vi "Computer GPS.vi"() -> ()   [LabVIEW 2009]
uses:
  UDP3-GPS, INS/UDP3rtglob.vi
  <instrlib>/u-blox 5 Series/u-blox 5 Series.lvlib
panel:
  out "output cluster":cluster{"Latitude":dbl, "Longitude":dbl}
  out "Valid Satalites":bool
  in  "stop":bool
  in  "Reset (False)":bool
  in  "VISA resource name":refnum<visa-resource-name>
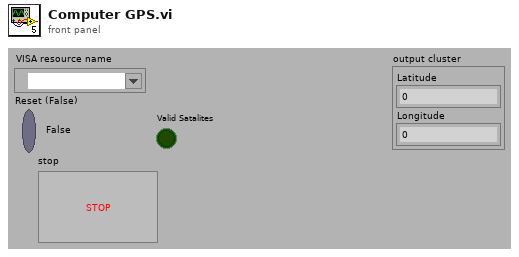
[diagram p1: front panel]
types:
  T1 = cluster{"Timestamp":timestamp, "Latitude":dbl, "Longitude":dbl}[]
  T2 = cluster{"Timestamp":timestamp, "Latitude":dbl, "Longitude":dbl}
  T3 = cluster{cluster{"Latitude":dbl, "Longitude":dbl}, cluster{dbl, dbl, dbl, dbl}}
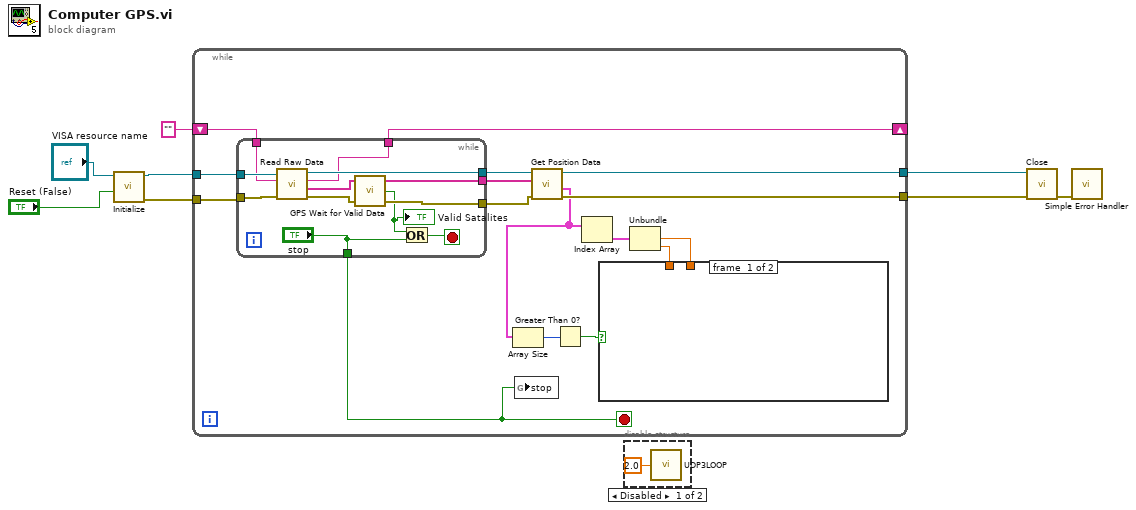
[diagram p0: block diagram]
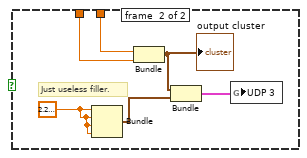
[diagram p3: hidden frame]
diagram:
  n1 = call <instrlib>:"Initialize.vi"("Reset (False)"="Reset (False)", "VISA resource name"="VISA resource name") -> ("error out"=w4:errorcluster, "VISA resource name out"=w5:refnum<visa-resource-name>)  [unwired: 8 in]
  n2 = while {
    shift-right: [w21] -> _
    shift-left: "" ("Remaining Partial Sentence") -> [w24]
    tunnel: w5 -> [w23]
    tunnel: w4 -> [w22]
    tunnel: [w15] -> w2
    tunnel: [w14] -> w3
    stop <- w9 stop-if-true
    n3 = while {
      tunnel: [w42] -> w20
      tunnel: w23 -> [w41]
      tunnel: w22 -> [w40]
      tunnel: w24 -> [w38]
      tunnel: [w35] -> w19
      tunnel: ["stop"] -> w9
      tunnel: [w34] -> w18
      tunnel: [w33] -> w21
      stop <- w39 stop-if-true
      n4 = call <instrlib>:"Read Raw Data.vi"("error in (no error)"=w40, "Previous Partial Sentence"=w38, "VISA resource name"=w41) -> ("error out"=w37:errorcluster, "Complete NMEA Sentences"=w36:string[], "Remaining Partial Sentence"=w33:string, "VISA resource name out"=w42:refnum<visa-resource-name>)  [unwired: 5 in]
      n5 = call "GPS Wait for Valid Data.vi"("error in (no error)"=w37, "Completed NMEA Sentences"=w36) -> ("error out"=w34:errorcluster, "Valid Data"=w32:bool, "Complete NMEA Sentences (Copy)"=w35:string[])  [unwired: 1 in]
      "Valid Satalites" <- w32
      n6 = Or(x=w32, y="stop") -> (x .or. y?=w39:bool)
    }
    n7 = global write "UDP3rtglob.vi" "stop"(w9) -> ()
    n8 = call <instrlib>:"Get Position Data.vi"("error in (no error)"=w18, "Complete NMEA Sentences"=w19, "VISA resource name"=w20) -> ("error out"=w14:errorcluster, "Position Data"=w10:T1, "VISA resource name out"=w15:refnum<visa-resource-name>)  [unwired: 5 in, 1 out]
    n9 = Array Size(array=w10) -> (size(s)=w17:i32)
    n10 = Greater Than 0?(x=w17) -> (x > 0?=w11:bool)
    n11 = Index Array(array=w10) -> (element=w16:T2)  [unwired: 1 in]
    n12 = Unbundle(w16) -> ("Latitude"=w12:dbl, "Longitude"=w13:dbl)  [unwired: 1 out]
    n13 = case shown="True" w11 {
      tunnel: w13 -> [_ w27]
      tunnel: w12 -> [_ w26]
      frame #0 {
      }
      frame #1 {
        w28 = 2.220446049250313e-16
        # "Just useless filler."
        n14 = Bundle(w28, w28, w28, w28) -> (w29:cluster{dbl, dbl, dbl, dbl})  [unwired: 1 in]
        n15 = Bundle("Latitude"=w26, "Longitude"=w27) -> (w30:cluster{"Latitude":dbl, "Longitude":dbl})  [unwired: 1 in]
        "output cluster" <- w30
        n16 = Bundle(w30, w29) -> (w25:T3)  [unwired: 1 in]
        n17 = global write "UDP3rtglob.vi" "UDP 3"(w25) -> ()
      }
    }
  }
  n18 = disable-structure shown="Disabled" {
    frame #0 {
      n19 = call "UDP3LOOP.vi"("Frequency, in Hz"=2.0) -> ()
    }
    frame #1 {
    }
  }
  n20 = call <instrlib>:"Close.vi"("error in (no error)"=w3, "VISA resource name"=w2) -> ("error out"=w1:errorcluster)  [unwired: 9 in]
  n21 = call <vilib>:"Simple Error Handler.vi"("error in (no error)"=w1) -> ()  [unwired: 4 in, 5 out]
